vi "remote.vi"() -> (2 "Caller string":string, 3 "Remote Call":bool, 5 "call chain":string[](array[string]))   [LabVIEW 2015]
doc: "Try to determine if the calling VI has been called locally or via VI server."
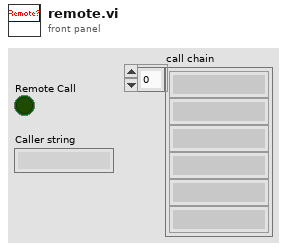
[diagram p1: front panel]
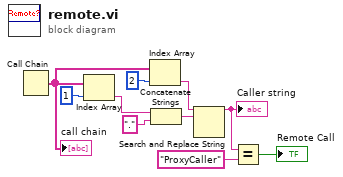
[diagram p0: block diagram]
diagram:
  n1 = Call Chain() -> (call chain=w4:string[])
  "call chain" <- w4
  n2 = Index Array(array=w4, index=1) -> (element=w6:string)
  n3 = Index Array(array=w4, index=2) -> (element=w2:string)
  n4 = Concatenate Strings(w6, "." ("string")) -> (w7:string)
  n5 = Search and Replace String(input string=w2, search string=w7) -> (result string=w8:string)  [unwired: 6 in, 3 out]
  "Caller string" <- w8
  n6 = Equal?(x=w8, y="ProxyCaller") -> (x = y?=→"Remote Call":bool)
